vi "指令规范.vi"(9 "参数":string, 10 "指令":T1, 11 "VISA资源名称":refnum<visa-resource-name>="COM3") -> (2 "响应":string)   [LabVIEW 2015]
uses:
  Program Files/National Instruments/LabVIEW 2015/examples/Instrument IO/Serial/support/Serial - Settings.ctl
  <vilib>/Instr/_visa.llb/VISA Configure Serial Port (Instr).vi
panel:
  in  "读取前延时(ms)":u32=500
  in  "串口设置":T2={"波特率"=115200, "数据比特"=8, "奇偶"=enum."None", "停止位"=10, "流控制"=0} {"流控制" items=["无"=0, "XON/XOFF"=1, "RTS/CTS"=2, "DTR/DSR"=4]; "停止位" items=["1.0"=10, "1.5"=15, "2.0"=20]; "数据比特" min=5 max=8 step=1; "波特率" items=["75"=75, "110"=110, "134"=134, "150"=150, "300"=300, "600"=600, "1200"=1200, "1800"=1800, "2400"=2400, "4800"=4800, "7200"=7200, "9600"=9600, "14400"=14400, "19200"=19200, "28800"=28800, "38400"=38400, "56000"=56000, "57600"=57600, "115200"=115200, "128000"=128000, "230400"=230400]}
  out "读取的字节":u32
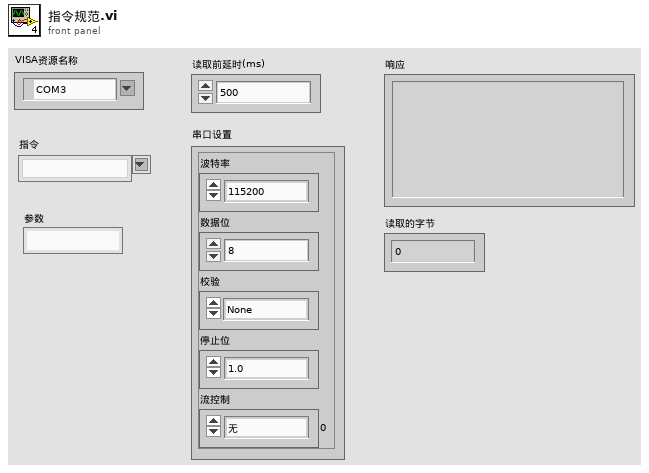
[diagram p1: front panel]
types:
  T1 = typedef "指令.ctl" = string
  T2 = typedef "Serial - Settings.ctl" = cluster{"波特率":u32, "数据比特":u16, "奇偶":enum16{"None", "Odd", "Even", "Mark", "Space"}, "停止位":u16, "流控制":u16}
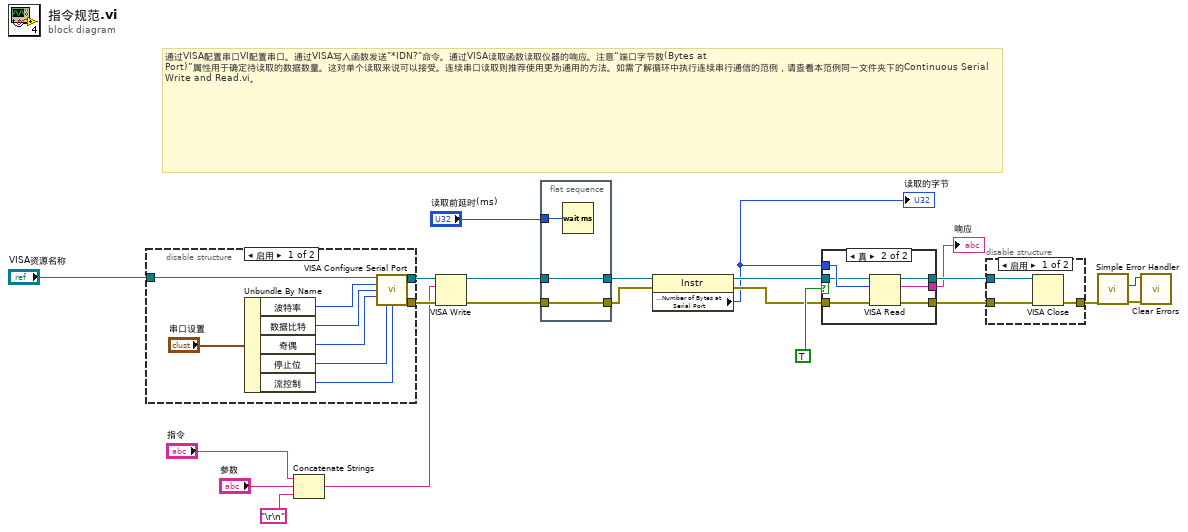
[diagram p0: block diagram]
diagram:
  # "通过VISA配置串口VI配置串口。通过VISA写入函数发送\"*IDN?\"命令。通过VISA读取函数读取仪器的响应。注意“端口字节数(Bytes at Port)”属性用于确定待读取的数据数量。这对单个读取来说可以接受。连续串口读取则推荐使用更为通用的方法。如需了解循环中执行连续串行通信的范例，请查看本范例同一文件夹下的Continuous Serial Write and Read.vi。"
  n1 = disable-structure shown="启用" {
    disable-tunnel: "VISA资源名称" -> [w31 w32]
    disable-tunnel: [w30 _] -> w21
    disable-tunnel: [w29 w32] -> w20
    frame Enabled {
      n2 = Unbundle By Name("串口设置") -> ("波特率"=w27:u32, "数据比特"=w26:u16, "奇偶"=w25:enum16{"None", "Odd", "Even", "Mark", "Space"}, "停止位"=w24:u16, "流控制"=w23:u16)
      n3 = call-poly "VISA Configure Serial Port"("VISA resource name"=w31, "baud rate (9600)"=w27, "data bits (8)"=w26, "parity (0:none)"=w25, "stop bits (10: 1 bit)"=w24, "flow control (0:none)"=w23) -> ("VISA resource name out"=w29:refnum<visa-resource-name>, "error out"=w30:errorcluster)  [unwired: 3 in, 5 out]
    }
    frame Disabled {
    }
  }
  n4 = Concatenate Strings("指令", "参数", "\r\n") -> (w1:string)
  n5 = VISA Write(VISA resource name=w20, write buffer=w1, error in (no error)=w21) -> (VISA resource name out=w12:refnum<visa-resource-name>, error out=w11:errorcluster)  [unwired: 1 out]
  n6 = flat-sequence {
    tunnel: w11 -> [w34]
    tunnel: [w34] -> w8
    tunnel: w12 -> [w33]
    tunnel: [w33] -> w9
    tunnel: "读取前延时(ms)" -> [w35]
    frame #0 {
      n7 = Wait (ms)(milliseconds to wait=w35) -> ()  [unwired: 1 out]
    }
  }
  n8 = property class="Instr"(reference=w9, error in=w8) -> (reference out=w7:refnum<visa-resource-name>, error out=w6:errorcluster, "Serial Settings:Number of Bytes at Serial Port"=w5:u32)
  "读取的字节" <- w5
  n9 = case shown="真" TRUE ("读指令") {
    tunnel: [w36 w43] -> w19
    tunnel: [w37 w42] -> w18
    tunnel: [_ w41] -> w16
    tunnel: w5 -> [_ w40]
    tunnel: w7 -> [w37 w39]
    tunnel: w6 -> [w36 w38]
    frame False {
    }
    frame True {
      n10 = VISA Read(VISA resource name=w39, byte count=w40, error in (no error)=w38) -> (VISA resource name out=w42:refnum<visa-resource-name>, read buffer=w41:string, error out=w43:errorcluster)  [unwired: 1 out]
    }
  }
  "响应" <- w16
  n11 = disable-structure shown="启用" {
    disable-tunnel: w19 -> [w46 w47]
    disable-tunnel: w18 -> [w45 _]
    disable-tunnel: [w44 w47] -> w17
    frame Enabled {
      n12 = VISA Close(VISA resource name=w45, error in (no error)=w46) -> (error out=w44:errorcluster)
    }
    frame Disabled {
    }
  }
  n13 = call <vilib>:"Simple Error Handler.vi"("error in (no error)"=w17) -> ("code out"=w13:i32, "error out"=w14:errorcluster)  [unwired: 1 in, 6 out]
  n14 = call <vilib>:"Clear Errors.vi"("error in (no error)"=w14, "specific error code to clear (0: all)"=w13) -> ()  [unwired: 4 in, 2 out]
